vi "beginPrepareGoalKickEnemyPlayVSS.vi"(8 "error in (no error)":errorcluster, 10 "Game in":refnum<class "Game.lvclass">, 11 "PrepareGoalKickEnemyPlayVSS in":refnum<class "PrepareGoalKickEnemyPlayVSS.lvclass">) -> (0 "error out":errorcluster, 2 "Boolean":bool, 3 "PrepareGoalKickEnemyPlayVSS out":refnum<class "PrepareGoalKickEnemyPlayVSS.lvclass">)   [LabVIEW 2023, in "PrepareGoalKickEnemyPlayVSS.lvclass"]
uses:
  PrepareGoalKickEnemyPlayVSS.lvclass
  Game_class/Game.lvclass
  Command.ctl
  Game_class/Game.lvclass/Game.ctl
  Game_class/Read Referee.vi
  Referee_class/Referee.lvclass
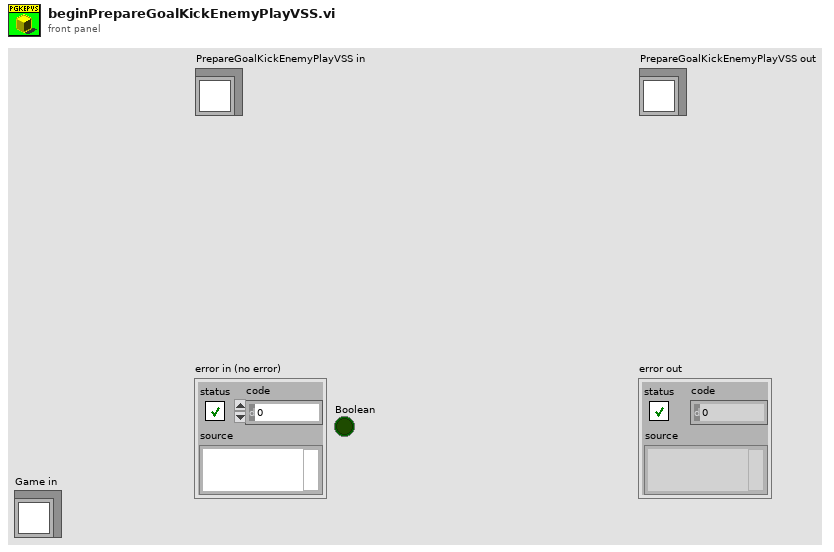
[diagram p1: front panel]
types:
  T1 = typedef "Command.ctl" = enum16{"AUTO", "GAME_ON", "STOP", "HALT", "KICKOFF_ALLY", "KICKOFF_ENEMY", "FREE_BALL", "GOAL_KICK_ENEMY", "GOAL_KICK_ALLY", "PENALTY_KICK_ENEMY", "PENALTY_KICK_ALLY", "FREE_KICK"}
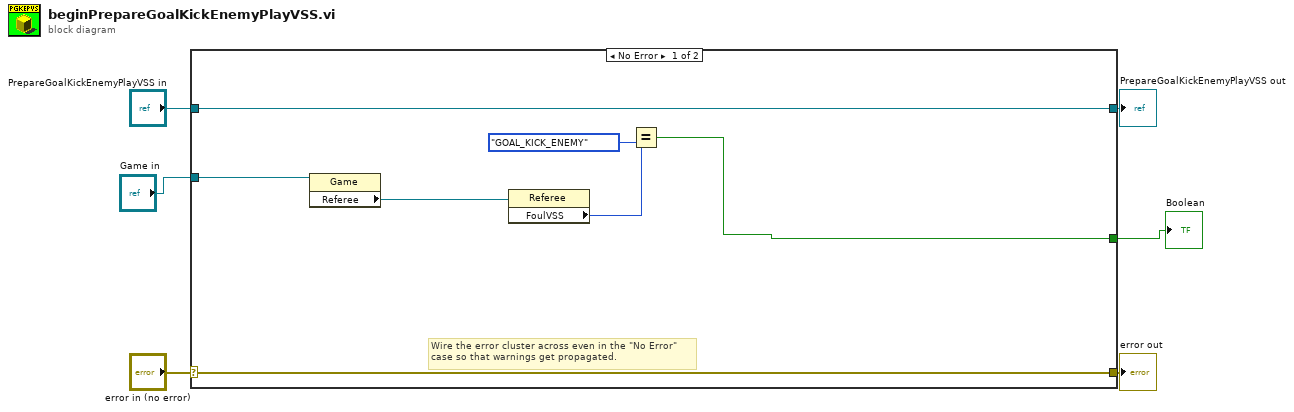
[diagram p0: block diagram]
diagram:
  n1 = case shown="No Error" "error in (no error)" {
    selector: "error in (no error)" -> [w12 w15]
    tunnel: [w12 w15] -> w5
    tunnel: [w13 w14] -> w3
    tunnel: "PrepareGoalKickEnemyPlayVSS in" -> [w13 w14]
    tunnel: "Game in" -> [w9 _]
    tunnel: [w7 _] -> w1
    frame No Error {
      # "Wire the error cluster across even in the \"No Error\"\ncase so that warnings get propagated."
      n2 = property class="Game"(reference=w9) -> ("Referee"=w11:refnum<class "Referee.lvclass">)  [unwired: 1 in, 2 out]
      n3 = property class="Referee"(reference=w11) -> ("FoulVSS"=w10:T1)  [unwired: 1 in, 2 out]
      n4 = Equal?(x=w10, y=Command."GOAL_KICK_ENEMY") -> (x = y?=w7:bool)
    }
    frame Error {
    }
  }
  "error out" <- w5
  "PrepareGoalKickEnemyPlayVSS out" <- w3
  "Boolean" <- w1
